vi "Configure Interactively.vi"(8 "error in (no error)":errorcluster, 10 "Parent Window":refnum<class "Window.lvclass">, 11 "Device in":refnum<class "Device.lvclass">) -> (0 "error out":errorcluster, 2 "Updated":bool, 3 "Device out":refnum<class "Device.lvclass">)   [LabVIEW 2015, in "IBEX Device.lvlib" / "Device.lvclass"]
doc: "Provides an interactive dialog for configuring the Device."
uses:
  Device.lvclass
  Window/Window.lvclass
panel:
  # "<Title>"
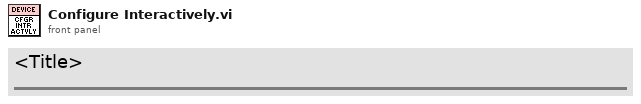
[diagram p1: front panel]
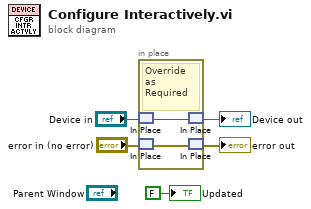
[diagram p0: block diagram]
diagram:
  n1 = in-place {
    # "Override as Required"
    n2 = in-place-match #1("Device in") -> (w6:refnum<class "Device.lvclass">)
    n3 = in-place-match #2("error in (no error)") -> (w7:errorcluster)
    n4 = in-place-match #1(w6) -> (→"Device out":refnum<class "Device.lvclass">)
    n5 = in-place-match #2(w7) -> (→"error out":errorcluster)
  }
  "Updated" <- FALSE
